vi "Shutdown.vi"(8 "error in (no error)":errorcluster) -> (0 "error out":errorcluster)   [LabVIEW 2015, in "App Config.lvlib"]
uses:
  App Config.lvlib
  FGV Action.ctl
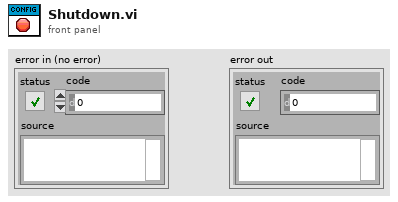
[diagram p1: front panel]
types:
  T1 = typedef "App Config.lvlib/FGV Action.ctl" = enum16{"Read", "Write"}
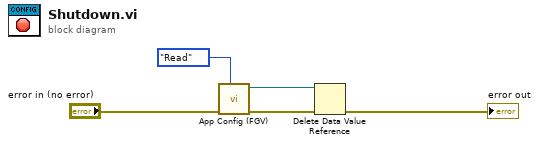
[diagram p0: block diagram]
diagram:
  n1 = call "App Config (FGV).vi"("Action (Read)"=FGV_Action."Read", "error in (no error)"="error in (no error)") -> ("error out"=w3:errorcluster, "DVR Out"=w2:refnum<data-value>)  [unwired: 8 in]
  n2 = Delete Data Value Reference(data value reference=w2, error in=w3) -> (error out=→"error out":errorcluster)  [unwired: 1 out]
